vi "LESO_read.vi"(8 "error in (no error)":errorcluster, 9 "Bytes To Read":u32, 11 "Handle in":u32) -> (0 "error out":errorcluster, 1 "Read Data":u8[](array[numeric]), 2 "FT_Status":u32(ring) items=["FT_OK", "FT_INVALID_HANDLE", "FT_DEVICE_NOT_FOUND", "FT_DEVICE_NOT_OPENED", "FT_IO_ERROR", "FT_INSUFFICIENT_RESOURCES", "FT_INVALID_PARAMETER", "FT_INVALID_BAUD_RATE", "FT_DEVICE_NOT_OPENED_FOR_ERASE", "FT_DEVICE_NOT_OPENED_FOR_WRITE", "FT_FAILED_TO_WRITE_DEVICE", "FT_EEPROM_READ_FAILED", "FT_EEPROM_WRITE_FAILED", "FT_EEPROM_ERASE_FAILED", "FT_EEPROM_NOT_PRESENT", "FT_EEPROM_NOT_PROGRAMMED", "FT_INVALID_ARGS", "FT_NOT_SUPPORTED", "FT_OTHER_ERROR"], 3 "Handle Out":u32, 4 "Bytes Read":u32)   [LabVIEW 2012]
doc: "Принимает массив данных с устройства."
uses:
  FTD2XX.dll
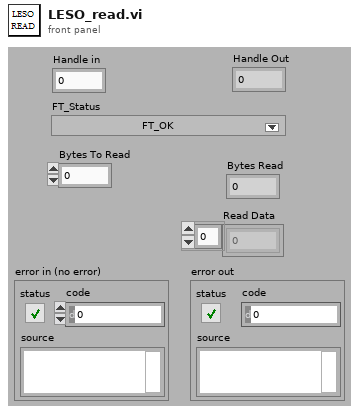
[diagram p1: front panel]
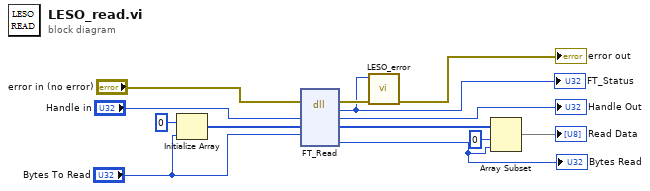
[diagram p0: block diagram]
diagram:
  n1 = Initialize Array(u8 0 ("element"), "Bytes To Read") -> (w12:u8[])
  n2 = dll-call lib="FTD2XX.dll" fn="FT_Read"(error in="error in (no error)", "Handle"="Handle in", "Buffer"=w12, "BytesToRead"="Bytes To Read") -> (error out=w5:errorcluster, "FT_Status"=w4:u32, "Handle"=→"Handle Out":u32, "Buffer"=w9:u8[], "BytesReturned"=w7:u32)  [unwired: 4 in, 1 out]
  "FT_Status" <- w4
  "Bytes Read" <- w7
  n3 = call "LESO_error.vi"("error in"=w5, "FT_Status"=w4) -> ("error out"=→"error out":errorcluster)  [unwired: 9 in]
  n4 = Array Subset(array=w9, index=0, length=w7) -> (→"Read Data":u8[])
